vi "ExampleReader.vi"() -> ()   [LabVIEW 2011]
uses:
  Reader/readType.ctl
  0x2 Typedefs/RIO-OCU update controls.ctl
  2-Think/2 Typedefs/generalized sensor status.ctl
  2-Think/2 Typedefs/indicator LED.ctl
  2-Think/2 Typedefs/generalized actuator status.ctl
  2-Think/2 Typedefs/Which Boat.ctl
  2-Think/2 Typedefs/robot velocity.ctl
  2-Think/2 Typedefs/UTM Location.ctl
  2-Think/2 Typedefs/heading.ctl
  2-Think/2 Typedefs/rate of turn.ctl
  2-Think/2 Typedefs/pitch and roll.ctl
  2-Think/2 Typedefs/apparent wind.ctl
  2-Think/2 Typedefs/apparent wind speed.ctl
  2-Think/2 Typedefs/apparent wind direction.ctl
  2-Think/2 Typedefs/Velocity.ctl
  2-Think/2 Typedefs/absolute wind direction.ctl
  2-Think/2 Typedefs/absolute wind speed.ctl
  2-Think/2 Typedefs/absolute water current vector.ctl
  2-Think/2 Typedefs/rudder angle.ctl
  2-Think/2 Typedefs/sail setpt.ctl
  0x2 Typedefs/manual override.ctl
  2-Think/2 Typedefs/setpoints to boat.ctl
  0x2 Typedefs/Current Waypoint.ctl
  2-Think/2 Globals/2 Global.vi
  Reader/NetworkStreamReader.lvclass
panel:
  out "Iteration Time Stamp":timestamp
  out "OCU Time Stamp":timestamp
  in  "stop":bool
  out "Monitored Items from RIO":T1 {"Robot Pitch/Roll"."Roll" format="%05.1f"; "Robot Pitch/Roll"."Pitch" format="%05.1f"; "Robot\nRate of Turn" format="%05.1f"; "Robot\nHeading" format="%05.1f"; "Robot UTM Location"."North" format="%#_10f"; "Robot UTM Location"."East" format="%#_8f"}
  in  "Read Type":T23=enum."Most current"
  in  "Loop delay (ms)":u32
  out "element":variant
  out "data":i32
  # "Note: writer is running at 50 ms"
  # "How Am I?"
  # "Where Am I?"
  # "Path Planning"
  # "From Planning Functions"
  # "(this is not a cluster because subitems\nare generated in parallel code)"
  # "What's Around Me?"
  # "As Measured"
  # "As Measured"
  # "Loop Rates"
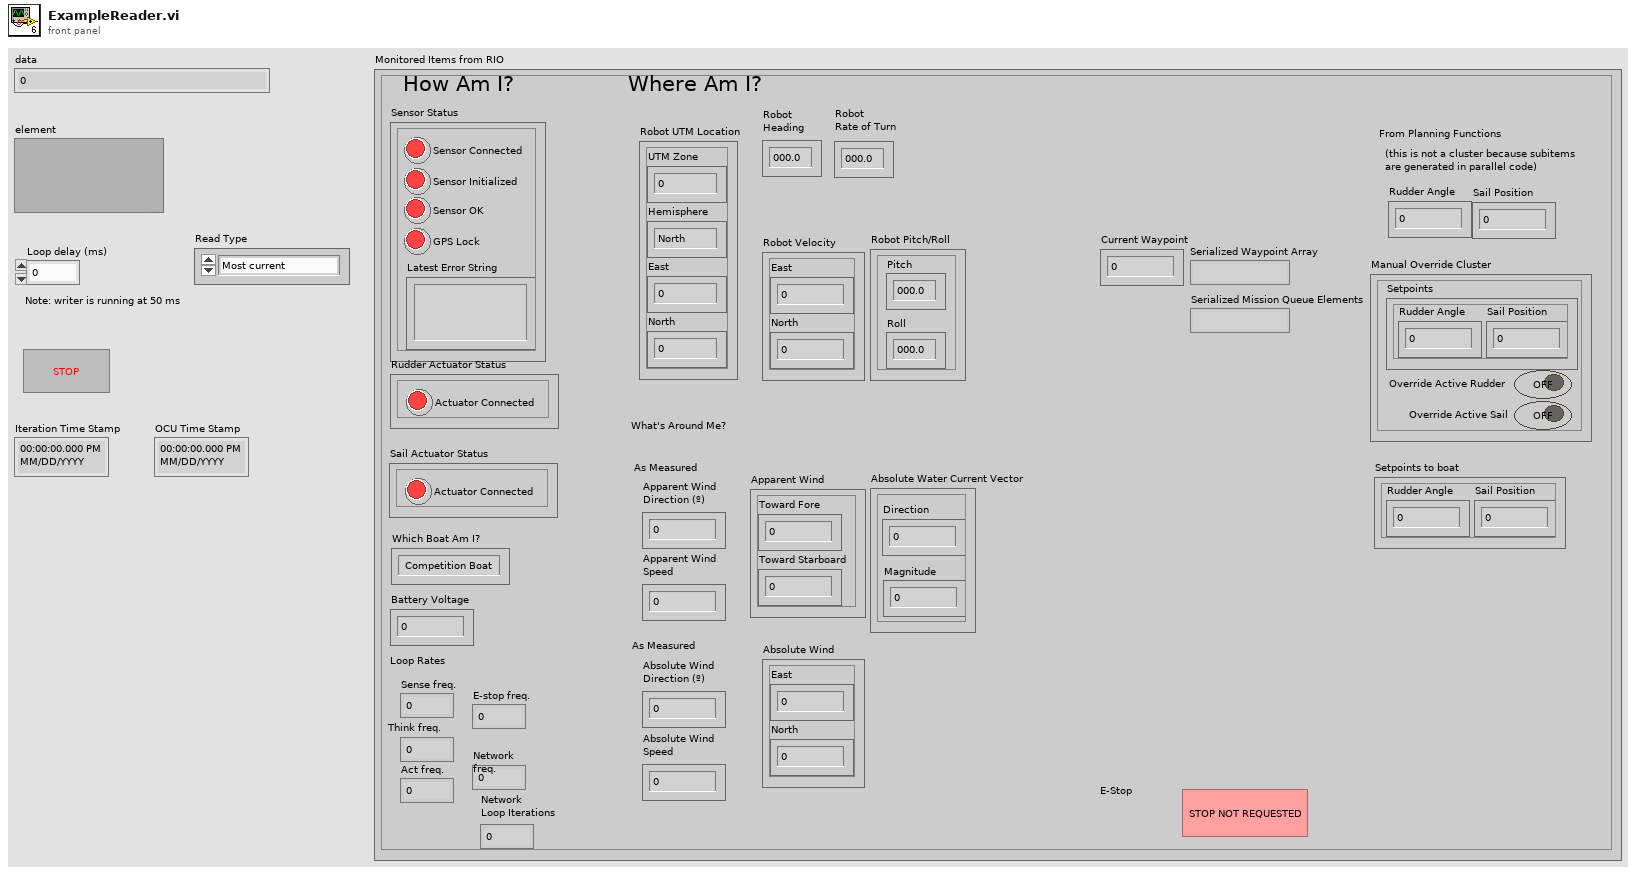
[diagram p1: front panel]
types:
  T1 = typedef "RIO-OCU update controls.ctl" = cluster{"Sensor Status":T2, "Battery Voltage":dbl, "Rudder Actuator Status":T4, "Sail Actuator Status":T4, "Which Boat Am I?":T5, "Robot Velocity":T6, "Robot UTM Location":T7, "Robot\nHeading ":T8, "Robot\nRate of Turn":T9, "Robot Pitch/Roll":T10, "Apparent Wind":T11, "Apparent Wind\nSpeed":T12, "Apparent Wind\nDirection (º)":T13, "Absolute Wind":T14, "Absolute Wind\nDirection (º)":T15, "Absolute Wind\nSpeed":T16, "Absolute Water Current Vector":T17, "Rudder Angle":T18, "Sail Position":T19, "Manual Override Cluster":T20, "Setpoints to boat":T21, "Current Waypoint":T22, "Think freq.":dbl, "Sense freq.":dbl, "Act freq.":dbl, "E-stop freq.":dbl, "Network \nfreq.":dbl, "Network \nLoop Iterations":i64, "E-Stop":bool, "Serialized Waypoint Array":string, "Serialized Mission Queue Elements":string}
  T2 = typedef "generalized sensor status.ctl" = cluster{"Sensor Connected":T3, "Sensor Initialized":T3, "Sensor OK":T3, "Latest Error String":string, "GPS Lock":T3}
  T3 = typedef "indicator LED.ctl" = bool
  T4 = typedef "generalized actuator status.ctl" = cluster{"Actuator Connected":T3}
  T5 = typedef "Which Boat.ctl" = enum16{"Competition Boat", "Small RC", "Simulation"}
  T6 = typedef "robot velocity.ctl" = cluster{"East":dbl, "North":dbl}
  T7 = typedef "UTM Location.ctl" = cluster{"UTM Zone":dbl, "Hemisphere":enum16{"North", "South"}, "East":dbl, "North":dbl}
  T8 = typedef "heading.ctl" = dbl
  T9 = typedef "rate of turn.ctl" = dbl
  T10 = typedef "pitch and roll.ctl" = cluster{"Pitch":dbl, "Roll":dbl}
  T11 = typedef "apparent wind.ctl" = cluster{"Toward Fore":dbl, "Toward Starboard":dbl}
  T12 = typedef "apparent wind speed.ctl" = dbl
  T13 = typedef "apparent wind direction.ctl" = dbl
  T14 = typedef "Velocity.ctl" = cluster{"East":dbl, "North":dbl}
  T15 = typedef "absolute wind direction.ctl" = dbl
  T16 = typedef "absolute wind speed.ctl" = dbl
  T17 = typedef "absolute water current vector.ctl" = cluster{"Direction":T13, "Magnitude":T13}
  T18 = typedef "rudder angle.ctl" = dbl
  T19 = typedef "sail setpt.ctl" = dbl
  T20 = typedef "manual override.ctl" = cluster{"Override Active Rudder":bool, "Setpoints":T21, "Override Active Sail":bool}
  T21 = typedef "setpoints to boat.ctl" = cluster{"Sail Position":T19, "Rudder Angle":T18}
  T22 = typedef "Current Waypoint.ctl" = i32
  T23 = typedef "NetworkStreamReader.lvclass/readType.ctl" = enum16{"Next in buffer", "Most current"}
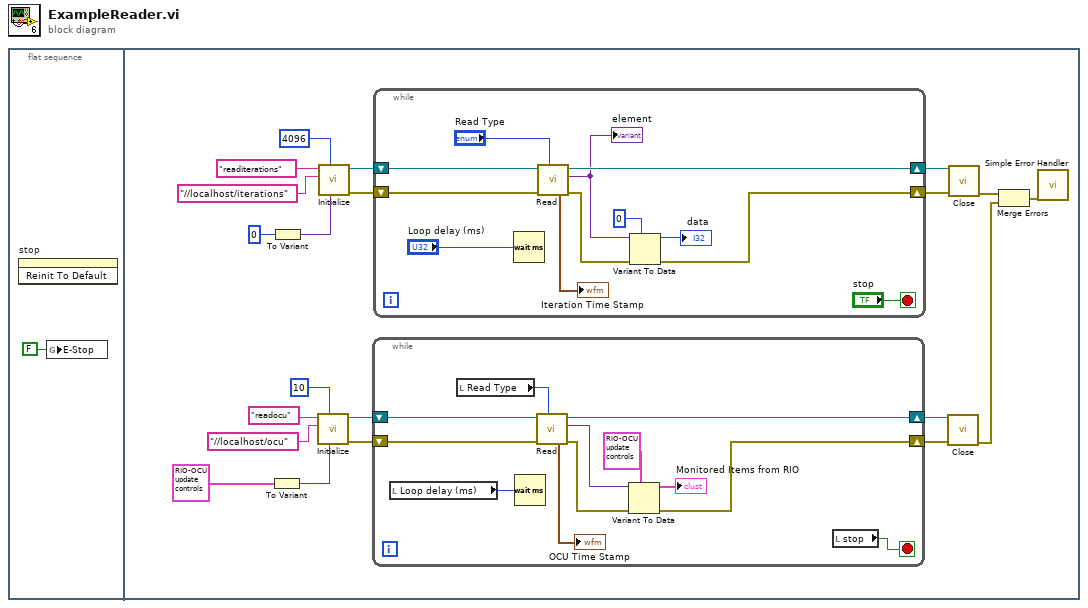
[diagram p0: block diagram]
diagram:
  n1 = flat-sequence {
    frame #0 {
      n2 = invoke on="stop" class="Bool (strict)" method="Reinit To Default"() -> ()  [unwired: 3 in, 3 out]
      n3 = global write "2 Global.vi" "E-Stop"(FALSE ("E-Stop")) -> ()
    }
    frame #1 {
      n4 = To Variant(anything=T1 {"Sensor Status"={"Sensor Connected"=FALSE, "Sensor Initialized"=FALSE, "Sensor OK"=FALSE, "Latest Error String"="", "GPS Lock"=FALSE}, "Battery Voltage"=0.0, "Rudder Actuator Status"={"Actuator Connected"=FALSE}, "Sail Actuator Status"={"Actuator Connected"=FALSE}, "Which Boat Am I?"=enum."Competition Boat", "Robot Velocity"={"East"=0.0, "North"=0.0}, "Robot UTM Location"={"UTM Zone"=0.0, "Hemisphere"=enum."North", "East"=0.0, "North"=0.0}, "Robot\nHeading "=0.0, "Robot\nRate of Turn"=0.0, "Robot Pitch/Roll"={"Pitch"=0.0, "Roll"=0.0}, "Apparent Wind"={"Toward Fore"=0.0, "Toward Starboard"=0.0}, "Apparent Wind\nSpeed"=0.0, "Apparent Wind\nDirection (º)"=0.0, "Absolute Wind"={"East"=0.0, "North"=0.0}, "Absolute Wind\nDirection (º)"=0.0, "Absolute Wind\nSpeed"=0.0, "Absolute Water Current Vector"={"Direction"=0.0, "Magnitude"=0.0}, "Rudder Angle"=0.0, "Sail Position"=0.0, "Manual Override Cluster"={"Override Active Rudder"=FALSE, "Setpoints"={"Sail Position"=0.0, "Rudder Angle"=0.0}, "Override Active Sail"=FALSE}, "Setpoints to boat"={"Sail Position"=0.0, "Rudder Angle"=0.0}, "Current Waypoint"=0, "Think freq."=0.0, "Sense freq."=0.0, "Act freq."=0.0, "E-stop freq."=0.0, "Network \nfreq."=0.0, "Network \nLoop Iterations"=0, "E-Stop"=FALSE, "Serialized Waypoint Array"="", "Serialized Mission Queue Elements"=""} ("Monitored Items from RIO")) -> (Variant=w15:variant)
      n5 = To Variant(anything=0) -> (Variant=w16:variant)
      n6 = call "Initialize.vi"("Default return"=w15, "reader buffer size"=10 ("writer buffer size"), "writer url"="//localhost/ocu", "reader name"="readocu") -> ("error out"=w10:errorcluster, "NetworkStreamWriter out"=w12:refnum<class "NetworkStreamReader.lvclass">)  [unwired: 5 in, 1 out]
      n7 = call "Initialize.vi"("Default return"=w16, "reader buffer size"=4096 ("writer buffer size"), "writer url"="//localhost/iterations", "reader name"="readiterations") -> ("error out"=w22:errorcluster, "NetworkStreamWriter out"=w20:refnum<class "NetworkStreamReader.lvclass">)  [unwired: 5 in, 1 out]
      n8 = while {
        shift-right: [w32] -> w14
        shift-left: w12 -> [w34]
        shift-right: [w27] -> w13
        shift-left: w10 -> [w33]
        stop <- w24 stop-if-true
        n9 = local read "Loop delay (ms)"() -> (w29:u32)
        n10 = local read "Read Type"() -> (w30:T23)
        n11 = Wait (ms)(milliseconds to wait=w29) -> ()  [unwired: 1 out]
        n12 = call "Read.vi"("Read Type"=w30, "error in (no error)"=w33, "NetworkStreamReader in"=w34) -> ("error out"=w28:errorcluster, "element"=w31:variant, "NetworkStreamReader out"=w32:refnum<class "NetworkStreamReader.lvclass">, "Time Stamp"=→"OCU Time Stamp":timestamp)  [unwired: 4 in, 1 out]
        n13 = Variant To Data(error in=w28, type=T1 {"Sensor Status"={"Sensor Connected"=FALSE, "Sensor Initialized"=FALSE, "Sensor OK"=FALSE, "Latest Error String"="", "GPS Lock"=FALSE}, "Battery Voltage"=0.0, "Rudder Actuator Status"={"Actuator Connected"=FALSE}, "Sail Actuator Status"={"Actuator Connected"=FALSE}, "Which Boat Am I?"=enum."Competition Boat", "Robot Velocity"={"East"=0.0, "North"=0.0}, "Robot UTM Location"={"UTM Zone"=0.0, "Hemisphere"=enum."North", "East"=0.0, "North"=0.0}, "Robot\nHeading "=0.0, "Robot\nRate of Turn"=0.0, "Robot Pitch/Roll"={"Pitch"=0.0, "Roll"=0.0}, "Apparent Wind"={"Toward Fore"=0.0, "Toward Starboard"=0.0}, "Apparent Wind\nSpeed"=0.0, "Apparent Wind\nDirection (º)"=0.0, "Absolute Wind"={"East"=0.0, "North"=0.0}, "Absolute Wind\nDirection (º)"=0.0, "Absolute Wind\nSpeed"=0.0, "Absolute Water Current Vector"={"Direction"=0.0, "Magnitude"=0.0}, "Rudder Angle"=0.0, "Sail Position"=0.0, "Manual Override Cluster"={"Override Active Rudder"=FALSE, "Setpoints"={"Sail Position"=0.0, "Rudder Angle"=0.0}, "Override Active Sail"=FALSE}, "Setpoints to boat"={"Sail Position"=0.0, "Rudder Angle"=0.0}, "Current Waypoint"=0, "Think freq."=0.0, "Sense freq."=0.0, "Act freq."=0.0, "E-stop freq."=0.0, "Network \nfreq."=0.0, "Network \nLoop Iterations"=0, "E-Stop"=FALSE, "Serialized Waypoint Array"="", "Serialized Mission Queue Elements"=""} ("Monitored Items from RIO"), Variant=w31) -> (data=→"Monitored Items from RIO":T1, error out=w27:errorcluster)
        n14 = local read "stop"() -> (w24:bool)
      }
      n15 = while {
        shift-right: [w44] -> w18
        shift-left: w20 -> [w46]
        shift-right: [w37] -> w19
        shift-left: w22 -> [w45]
        stop <- "stop" stop-if-true
        n16 = Wait (ms)(milliseconds to wait="Loop delay (ms)") -> ()  [unwired: 1 out]
        n17 = call "Read.vi"("Read Type"="Read Type", "error in (no error)"=w45, "NetworkStreamReader in"=w46) -> ("error out"=w38:errorcluster, "element"=w43:variant, "NetworkStreamReader out"=w44:refnum<class "NetworkStreamReader.lvclass">, "Time Stamp"=→"Iteration Time Stamp":timestamp)  [unwired: 4 in, 1 out]
        "element" <- w43
        n18 = Variant To Data(error in=w38, type=0, Variant=w43) -> (data=→"data":i32, error out=w37:errorcluster)
      }
      n19 = call "Close.vi"("error in (no error)"=w13, "NetworkStreamReader in"=w14) -> ("error out"=w8:errorcluster)  [unwired: 8 in, 1 out]
      n20 = call "Close.vi"("error in (no error)"=w19, "NetworkStreamReader in"=w18) -> ("error out"=w9:errorcluster)  [unwired: 8 in, 1 out]
      n21 = Merge Errors(w9, w8) -> (w7:errorcluster)
      n22 = call <vilib>:"Simple Error Handler.vi"("error in (no error)"=w7) -> ()  [unwired: 4 in, 5 out]
    }
  }
